vi "ajustement_lineaire.vi"(0 "Y":dbl[](array[numeric])) -> (1 "Best Linear Fit":dbl[](array[numeric]) caption="Meilleur ajustement linéaire", 2 "slope":dbl caption="pente")   [LabVIEW 2020]
uses:
  <vilib>/Analysis/6fits.llb/Curve Fitting Criteria.ctl
  <vilib>/Analysis/Matrix/Numeric/Conversions/Array To Matrix - RA.vi
  <vilib>/Analysis/NI_AALPro.lvlib
  <vilib>/Analysis/Matrix/NI_Matrix.lvlib
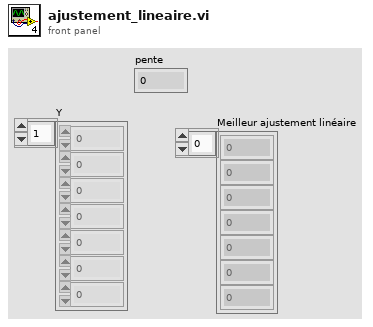
[diagram p1: front panel]
types:
  T1 = typedef "NI_AALPro.lvlib/Curve Fitting Criteria.ctl" = u16
  T2 = typedef "NI_Matrix.lvlib/RealMatrix.ctl" = dbl[][]
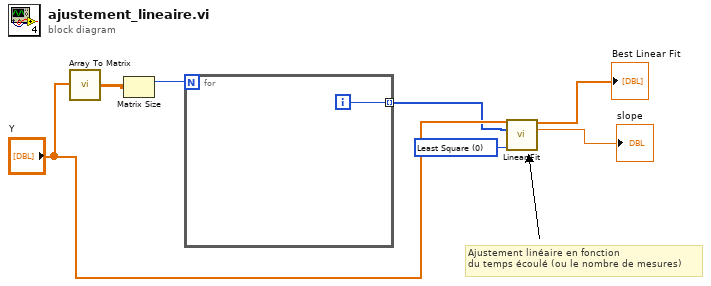
[diagram p0: block diagram]
diagram:
  w1 = T1 0 items=["Least Square", "Least Absolute Residual", "Bisquare"] ("method")
  # "Ajustement linéaire en fonction\ndu temps écoulé (ou le nombre de mesures)"
  n1 = call-poly <vilib>:"Array To Matrix.vi"("Real 1D Array"="Y") -> ("Real Matrix (Column Vector)"=w4:T2)
  n2 = Matrix Size(0:w4) -> (1:w5:i32)  [unwired: 1 out]
  n3 = for {
    N: w5 -> [_]
    tunnel: [w8] -> w2 mode=indexing
    i -> [w8]
  }
  n4 = call <vilib>:"Linear Fit.vi"("Y"="Y", "X"=w2, "method"=w1) -> ("Best Linear Fit"=→"Best Linear Fit":dbl[], "slope"=→"slope":dbl)  [unwired: 8 in, 3 out]
